vi "write_params.vi"(8 "error in (no error)":errorcluster, 10 "params":T1={"alpha"=0.999999999999999, "fit_prior"=TRUE, "class_prior"={"class_prior_type"="None", "class_prior_list"=[]}, "norm"=FALSE}, 11 "ComplementNB in":refnum<class "ComplementNB.lvclass">) -> (0 "error out":errorcluster, 3 "ComplementNB out":refnum<class "ComplementNB.lvclass">)   [LabVIEW 2020, in "ComplementNB.lvclass"]
uses:
  ComplementNB.lvclass
  Controls/complement_nb_params.ctl
  ComplementNB.lvclass/ComplementNB.ctl
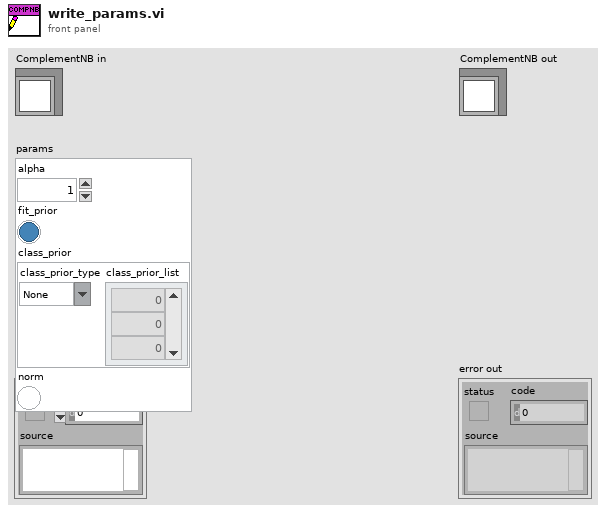
[diagram p1: front panel]
types:
  T1 = typedef "complement_nb_params.ctl" = cluster{"alpha":dbl, "fit_prior":bool, "class_prior":cluster{"class_prior_type":string, "class_prior_list":dbl[]}, "norm":bool}
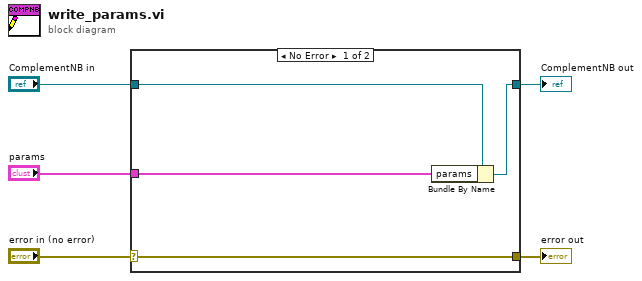
[diagram p0: block diagram]
diagram:
  n1 = case shown="No Error" "error in (no error)" {
    selector: "error in (no error)" -> [w9 w10]
    tunnel: [w9 w10] -> w4
    tunnel: [w7 w11] -> w2
    tunnel: "ComplementNB in" -> [w8 w11]
    tunnel: "params" -> [w6 _]
    frame No Error {
      n2 = Bundle By Name(cluster=w8, "params"=w6) -> (w7:refnum<class "ComplementNB.lvclass">)
    }
    frame Error {
    }
  }
  "error out" <- w4
  "ComplementNB out" <- w2
